vi "ZZZ Chroma 1905x Series Configure POP.vi"(0 "inst handle in":refnum<visa-resource-name>, 7 "error in":T1) -> (20 "inst handle out":refnum<visa-resource-name>, 23 "Identification":string, 27 "error out":T1)   [LabVIEW 2025]
doc: "Contact Chroma\nTEL: +886-2-2298-3855 \nTEL: +886-3-397-5788 \nFAX: +886-2-2298-3596\nFAX: +886-3-327-4703 \nURL: http://www.chromaate.com \nE-mail: chroma@chroma.com.tw"
uses:
  <instrlib>/Chroma 19052/Chroma 19052.lvlib
panel:
  in  "Step":dbl=1.0 min=1.0 max=99.0 step=1.0
  in  "Real Current Limit":dbl min=0.0 max=0.03 step=1e-06 format="%.2p"
  in  "Finished":bool
  in  "Configure":bool
  in  "Frequency":u16(ring)=1 items=["50", "60"]
  in  "Voltage Level IR":dbl=1000.0 min=100.0 max=1000.0 step=2.0
  in  "Hi Limit":dbl min=0.0 max=50000000000.0 step=10000.0 format="%.2p"
  in  "Low Limit":dbl=10000000.0 min=100000.0 max=50000000000.0 step=10000.0 format="%.2p"
  in  "ARC Limit":dbl min=0.0 max=0.015 step=1e-06 format="%.2p"
  in  "Test Time":dbl=3.0 min=0.0 max=999.0 step=0.1 format="%.1f"
  in  "Ramp Time":dbl min=0.0 max=999.0 step=0.1 format="%.1f"
  in  "Hi Limit":dbl=0.001 min=1e-06 max=0.03 step=1e-06 format="%.2p"
  in  "Low Limit":dbl min=0.0 max=0.03 step=1e-06 format="%.2p"
  in  "Voltage Level":dbl=1000.0 min=100.0 max=6000.0 step=2.0
  in  "Mode":u16(ring) items=["AC", "DC", "IR"]
  # "Configuration Screen"
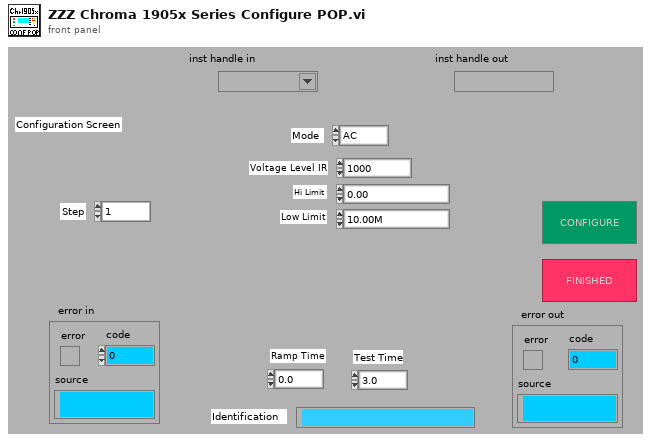
[diagram p1: front panel]
types:
  T1 = cluster{"error":bool, "code":i8, "source":string}
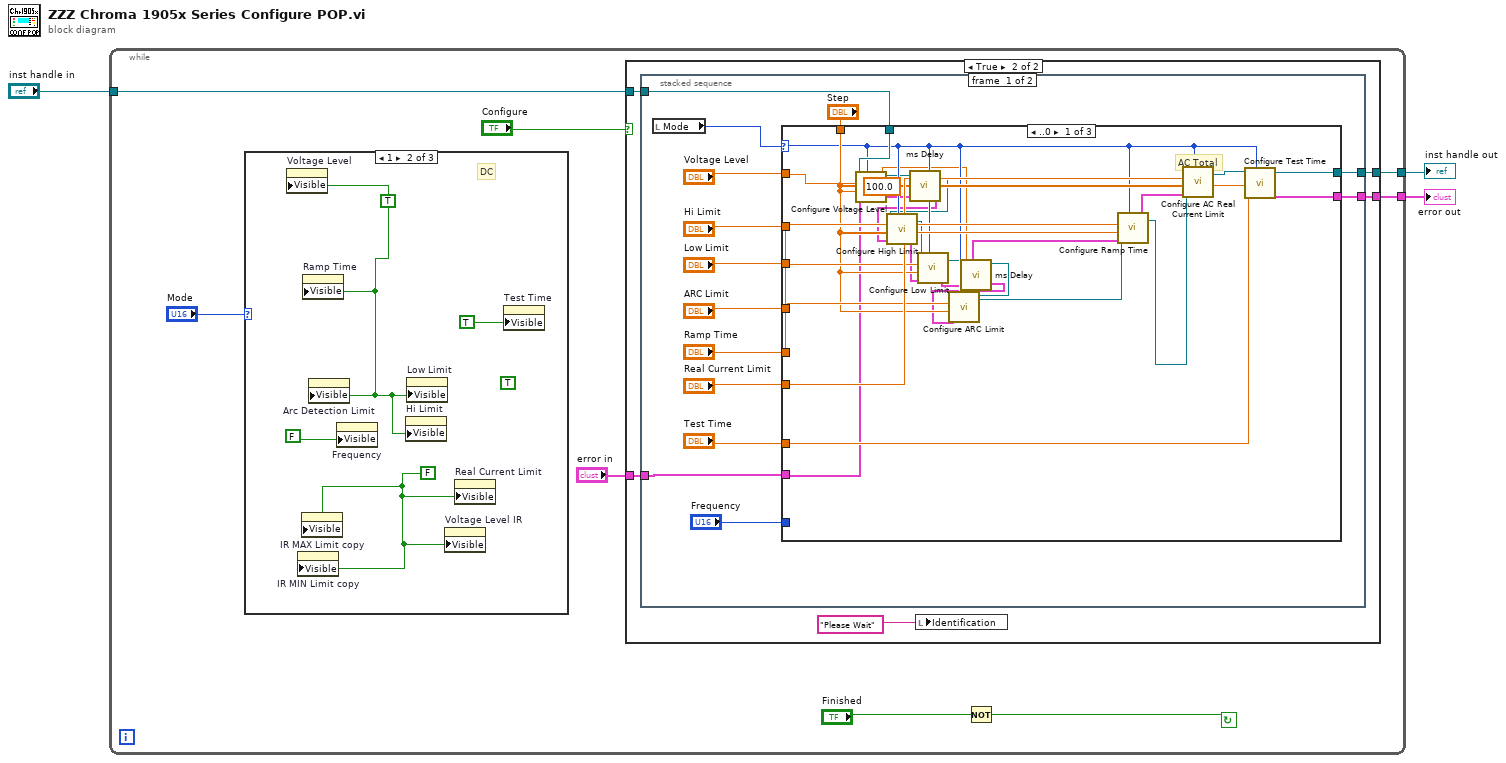
[diagram p0: block diagram]
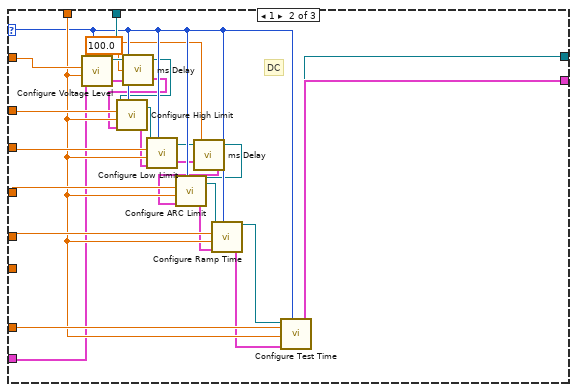
[diagram p3: hidden frame]
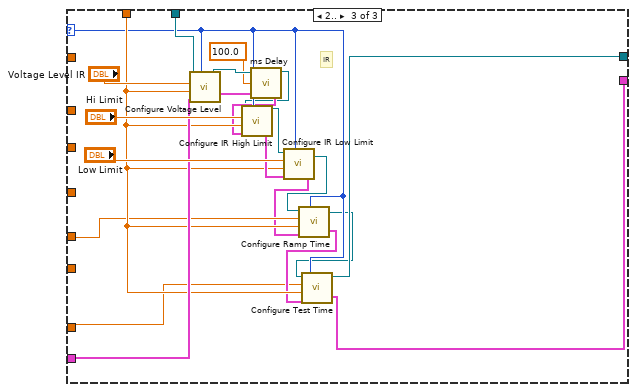
[diagram p4: hidden frame]
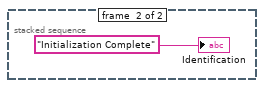
[diagram p5: hidden frame]
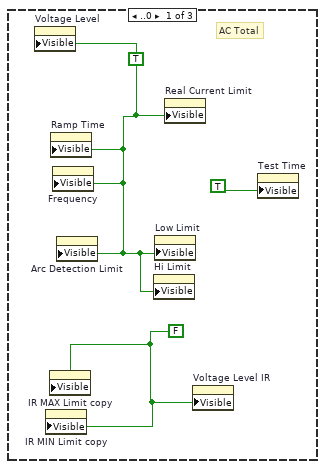
[diagram p6: hidden frame]
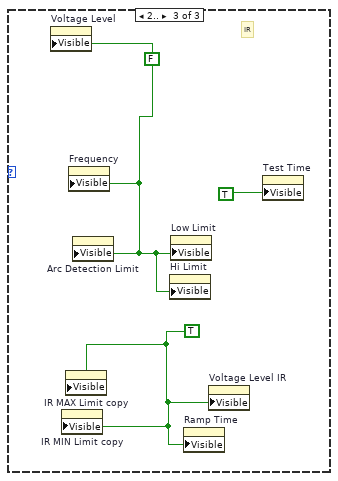
[diagram p7: hidden frame]
diagram:
  n1 = while {
    tunnel: "inst handle in" -> [w9]
    tunnel: [w10] -> w3
    tunnel: [w11] -> w2
    stop <- w7 continue-if-true
    n2 = case shown="1" "Mode" {
      frame ..0 {
        w113 = FALSE
        w112 = TRUE
        # "AC Total"
        n3 = property on="Voltage Level" class="DigNum (strict)"("Visible"=w112) -> ()  [unwired: 2 in, 2 out]
        n4 = property on="IR MIN Limit copy" class="DigNum (strict)"("Visible"=w113) -> ()  [unwired: 2 in, 2 out]
        n5 = property on="IR MAX Limit copy" class="DigNum (strict)"("Visible"=w113) -> ()  [unwired: 2 in, 2 out]
        n6 = property on="Ramp Time" class="DigNum (strict)"("Visible"=w112) -> ()  [unwired: 2 in, 2 out]
        n7 = property on="Frequency" class="Ring (strict)"("Visible"=w112) -> ()  [unwired: 2 in, 2 out]
        n8 = property on="Arc Detection Limit" class="DigNum (strict)"("Visible"=w112) -> ()  [unwired: 2 in, 2 out]
        n9 = property on="Hi Limit" class="DigNum (strict)"("Visible"=w112) -> ()  [unwired: 2 in, 2 out]
        n10 = property on="Low Limit" class="DigNum (strict)"("Visible"=w112) -> ()  [unwired: 2 in, 2 out]
        n11 = property on="Real Current Limit" class="DigNum (strict)"("Visible"=w112) -> ()  [unwired: 2 in, 2 out]
        n12 = property on="Voltage Level IR" class="DigNum (strict)"("Visible"=w113) -> ()  [unwired: 2 in, 2 out]
        n13 = property on="Test Time" class="DigNum (strict)"("Visible"=TRUE) -> ()  [unwired: 2 in, 2 out]
      }
      frame 1 {
        (unwired) TRUE
        w115 = FALSE
        w117 = TRUE
        # "DC"
        n14 = property on="Voltage Level" class="DigNum (strict)"("Visible"=w117) -> ()  [unwired: 2 in, 2 out]
        n15 = property on="IR MIN Limit copy" class="DigNum (strict)"("Visible"=w115) -> ()  [unwired: 2 in, 2 out]
        n16 = property on="IR MAX Limit copy" class="DigNum (strict)"("Visible"=w115) -> ()  [unwired: 2 in, 2 out]
        n17 = property on="Ramp Time" class="DigNum (strict)"("Visible"=w117) -> ()  [unwired: 2 in, 2 out]
        n18 = property on="Arc Detection Limit" class="DigNum (strict)"("Visible"=w117) -> ()  [unwired: 2 in, 2 out]
        n19 = property on="Frequency" class="Ring (strict)"("Visible"=FALSE) -> ()  [unwired: 2 in, 2 out]
        n20 = property on="Hi Limit" class="DigNum (strict)"("Visible"=w117) -> ()  [unwired: 2 in, 2 out]
        n21 = property on="Low Limit" class="DigNum (strict)"("Visible"=w117) -> ()  [unwired: 2 in, 2 out]
        n22 = property on="Voltage Level IR" class="DigNum (strict)"("Visible"=w115) -> ()  [unwired: 2 in, 2 out]
        n23 = property on="Real Current Limit" class="DigNum (strict)"("Visible"=w115) -> ()  [unwired: 2 in, 2 out]
        n24 = property on="Test Time" class="DigNum (strict)"("Visible"=TRUE) -> ()  [unwired: 2 in, 2 out]
      }
      frame 2.. {
        w119 = TRUE
        w120 = FALSE
        # "IR"
        n25 = property on="Voltage Level" class="DigNum (strict)"("Visible"=w120) -> ()  [unwired: 2 in, 2 out]
        n26 = property on="IR MIN Limit copy" class="DigNum (strict)"("Visible"=w119) -> ()  [unwired: 2 in, 2 out]
        n27 = property on="IR MAX Limit copy" class="DigNum (strict)"("Visible"=w119) -> ()  [unwired: 2 in, 2 out]
        n28 = property on="Frequency" class="Ring (strict)"("Visible"=w120) -> ()  [unwired: 2 in, 2 out]
        n29 = property on="Arc Detection Limit" class="DigNum (strict)"("Visible"=w120) -> ()  [unwired: 2 in, 2 out]
        n30 = property on="Hi Limit" class="DigNum (strict)"("Visible"=w120) -> ()  [unwired: 2 in, 2 out]
        n31 = property on="Low Limit" class="DigNum (strict)"("Visible"=w120) -> ()  [unwired: 2 in, 2 out]
        n32 = property on="Ramp Time" class="DigNum (strict)"("Visible"=w119) -> ()  [unwired: 2 in, 2 out]
        n33 = property on="Voltage Level IR" class="DigNum (strict)"("Visible"=w119) -> ()  [unwired: 2 in, 2 out]
        n34 = property on="Test Time" class="DigNum (strict)"("Visible"=TRUE) -> ()  [unwired: 2 in, 2 out]
      }
    }
    n35 = case shown="True" "Configure" {
      tunnel: w9 -> [w13 w18]
      tunnel: [w13 w17] -> w10
      tunnel: [w12 w16] -> w11
      tunnel: "error in" -> [w12 w15]
      frame False {
      }
      frame True {
        n36 = stacked-sequence {
          tunnel: w18 -> [w32 _]
          tunnel: w15 -> [w30 _]
          tunnel: [w22 _] -> w17
          tunnel: [w21 _] -> w16
          frame #0 {
            n37 = local read "Mode"() -> (w23:u16)
            n38 = case shown="..0" w23 {
              selector: w23 -> [w48 w78 w101]
              tunnel: w32 -> [w53 w81 w107]
              tunnel: "Test Time" -> [w55 w83 w99]
              tunnel: [w42 w73 w95] -> w22
              tunnel: w30 -> [w44 w75 w104]
              tunnel: [w43 w74 w96] -> w21
              tunnel: "Ramp Time" -> [w60 w88 w98]
              tunnel: "ARC Limit" -> [w59 w87 _]
              tunnel: "Low Limit" -> [w58 w86 _]
              tunnel: "Hi Limit" -> [w57 w85 _]
              tunnel: "Voltage Level" -> [w56 w84 _]
              tunnel: "Frequency" -> [_ _ _]
              tunnel: "Real Current Limit" -> [w61 _ _]
              tunnel: "Step" -> [w54 w82 w103]
              frame ..0 {
                w33 = 100.0 ("Time Delay S")
                # "AC Total"
                n39 = call <instrlib>:"Configure Voltage Level.vi"("VISA session copy"=w53, "Voltage Level"=w56, "Step"=w54, "error in"=w44, "Mode"=w48) -> ("VISA session"=w40:refnum<visa-resource-name>, "error out"=w41:T1)
                n40 = call <instrlib>:"ms Delay.vi"("error in"=w41, "Time Delay S"=w33, "inst handle in"=w40) -> ("error out"=w38:T1, "inst handle Out"=w39:refnum<visa-resource-name>)
                n41 = call <instrlib>:"Configure High Limit.vi"("VISA session copy"=w39, "Hi Limit"=w57, "Step"=w54, "error in"=w38, "Mode"=w48) -> ("VISA session"=w52:refnum<visa-resource-name>, "error out"=w47:T1)
                n42 = call <instrlib>:"Configure Low Limit.vi"("VISA session copy"=w52, "Low Limit"=w58, "Step"=w54, "error in"=w47, "Mode"=w48) -> ("VISA session"=w37:refnum<visa-resource-name>, "error out"=w36:T1)
                n43 = call <instrlib>:"ms Delay.vi"("error in"=w36, "Time Delay S"=w33, "inst handle in"=w37) -> ("error out"=w35:T1, "inst handle Out"=w34:refnum<visa-resource-name>)
                n44 = call <instrlib>:"Configure ARC Limit.vi"("VISA session copy"=w34, "ARC Limit"=w59, "Step"=w54, "error in"=w35, "Mode"=w48) -> ("VISA session"=w51:refnum<visa-resource-name>, "error out"=w46:T1)
                n45 = call <instrlib>:"Configure Ramp Time.vi"("VISA session copy"=w51, "Ramp Time"=w60, "Step"=w54, "error in"=w46, "Mode"=w48) -> ("VISA session"=w50:refnum<visa-resource-name>, "error out"=w45:T1)
                n46 = call <instrlib>:"Configure AC Real Current Limit.vi"("VISA session copy"=w50, "Real Current Limit"=w61, "Step"=w54, "error in"=w45, "Mode"=w48) -> ("VISA session"=w49:refnum<visa-resource-name>)  [unwired: 1 out]
                n47 = call <instrlib>:"Configure Test Time.vi"("VISA session copy"=w49, "Test Time"=w55, "Step"=w54, "Mode"=w48) -> ("VISA session"=w42:refnum<visa-resource-name>, "error out"=w43:T1)  [unwired: 1 in]
              }
              frame 1 {
                w64 = 100.0 ("Time Delay S")
                # "DC"
                n48 = call <instrlib>:"Configure Voltage Level.vi"("VISA session copy"=w81, "Voltage Level"=w84, "Step"=w82, "error in"=w75, "Mode"=w78) -> ("VISA session"=w72:refnum<visa-resource-name>, "error out"=w69:T1)
                n49 = call <instrlib>:"ms Delay.vi"("error in"=w69, "Time Delay S"=w64, "inst handle in"=w72) -> ("error out"=w70:T1, "inst handle Out"=w71:refnum<visa-resource-name>)
                n50 = call <instrlib>:"Configure High Limit.vi"("VISA session copy"=w71, "Hi Limit"=w85, "Step"=w82, "error in"=w70, "Mode"=w78) -> ("VISA session"=w80:refnum<visa-resource-name>, "error out"=w77:T1)
                n51 = call <instrlib>:"Configure Low Limit.vi"("VISA session copy"=w80, "Low Limit"=w86, "Step"=w82, "error in"=w77, "Mode"=w78) -> ("VISA session"=w68:refnum<visa-resource-name>, "error out"=w67:T1)
                n52 = call <instrlib>:"ms Delay.vi"("error in"=w67, "Time Delay S"=w64, "inst handle in"=w68) -> ("error out"=w65:T1, "inst handle Out"=w66:refnum<visa-resource-name>)
                n53 = call <instrlib>:"Configure ARC Limit.vi"("VISA session copy"=w66, "ARC Limit"=w87, "Step"=w82, "error in"=w65, "Mode"=w78) -> ("VISA session"=w79:refnum<visa-resource-name>, "error out"=w76:T1)
                n54 = call <instrlib>:"Configure Ramp Time.vi"("VISA session copy"=w79, "Ramp Time"=w88, "Step"=w82, "error in"=w76, "Mode"=w78) -> ("VISA session"=w62:refnum<visa-resource-name>, "error out"=w63:T1)
                n55 = call <instrlib>:"Configure Test Time.vi"("VISA session copy"=w62, "Test Time"=w83, "Step"=w82, "error in"=w63, "Mode"=w78) -> ("VISA session"=w73:refnum<visa-resource-name>, "error out"=w74:T1)
              }
              frame 2.. {
                # "IR"
                n56 = call <instrlib>:"Configure Voltage Level.vi"("VISA session copy"=w107, "Voltage Level"="Voltage Level IR", "Step"=w103, "error in"=w104, "Mode"=w101) -> ("VISA session"=w90:refnum<visa-resource-name>, "error out"=w93:T1)
                n57 = call <instrlib>:"ms Delay.vi"("error in"=w93, "Time Delay S"=100.0, "inst handle in"=w90) -> ("error out"=w92:T1, "inst handle Out"=w91:refnum<visa-resource-name>)
                n58 = call <instrlib>:"Configure IR High Limit.vi"("VISA session copy"=w91, "Hi Limit"="Hi Limit", "Step"=w103, "error in"=w92, "Mode"=w101) -> ("VISA session"=w105:refnum<visa-resource-name>, "error out"=w106:T1)
                n59 = call <instrlib>:"Configure IR Low Limit.vi"("VISA session copy"=w105, "Low Limit"="Low Limit", "Step"=w103, "error in"=w106, "Mode"=w101) -> ("VISA session"=w102:refnum<visa-resource-name>, "error out"=w97:T1)
                n60 = call <instrlib>:"Configure Ramp Time.vi"("VISA session copy"=w102, "Ramp Time"=w98, "Step"=w103, "error in"=w97, "Mode"=w101) -> ("VISA session"=w94:refnum<visa-resource-name>, "error out"=w100:T1)
                n61 = call <instrlib>:"Configure Test Time.vi"("VISA session copy"=w94, "Test Time"=w99, "Step"=w103, "error in"=w100, "Mode"=w101) -> ("VISA session"=w95:refnum<visa-resource-name>, "error out"=w96:T1)
              }
            }
          }
          frame #1 {
            "Identification" <- "Initialization Complete"
          }
        }
        n62 = local write "Identification"("Please Wait") -> ()
      }
    }
    n63 = Not(x="Finished") -> (.not. x?=w7:bool)
  }
  "error out" <- w2
  "inst handle out" <- w3
